vi "ciąg fibonacciego.vi"() -> ()   [LabVIEW 2020]
panel:
  in  "Określ ilość elementów ciągu fibonacciego":i32
  out "Ciąg fibonacciego do określonego powyżej elementu":string
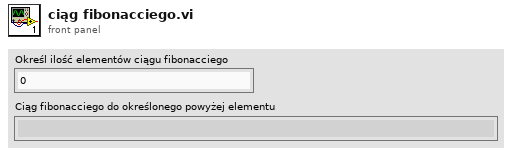
[diagram p1: front panel]
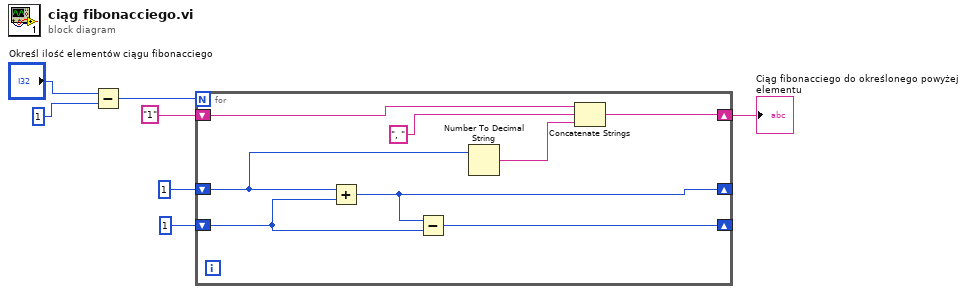
[diagram p0: block diagram]
diagram:
  n1 = Subtract(x="Określ ilość elementów ciągu fibonacciego", y=1) -> (x-y=w3:i32)
  n2 = for {
    N: w3 -> [_]
    shift-right: [w15] -> _
    shift-left: 1 -> [w10]
    shift-right: [w11] -> _
    shift-left: 1 -> [w8]
    shift-right: [w12] -> w4
    shift-left: "1" -> [w14]
    n3 = Add(x=w8, y=w10) -> (x+y=w11:i32)
    n4 = Subtract(x=w11, y=w10) -> (x-y=w15:i32)
    n5 = Number To Decimal String(number=w8) -> (decimal integer string=w9:string)  [unwired: 1 in]
    n6 = Concatenate Strings(w14, ", ", w9) -> (w12:string)
  }
  "Ciąg fibonacciego do określonego powyżej elementu" <- w4
